vi "GenSet_AE.vi"(7 "Enum":enum16{"READ", "WRITE"}(ring), 10 "General settings":T1={"Holo size (pixels)"=0, "Top hat radius"=0.5, "Number of modes"=0, "Bkg gradient X"=0.0, "Bkg gradient Y"=0.0, "Flat"=FALSE, "Mode Matrix"=0}) -> (2 "General settings Out":T1={"Holo size (pixels)"=0, "Top hat radius"=0.0, "Number of modes"=0, "Bkg gradient X"=0.0, "Bkg gradient Y"=-40.0, "Flat"=FALSE, "Mode Matrix"=0})   [LabVIEW 2014]
uses:
  Controls/SLM General Settings.ctl
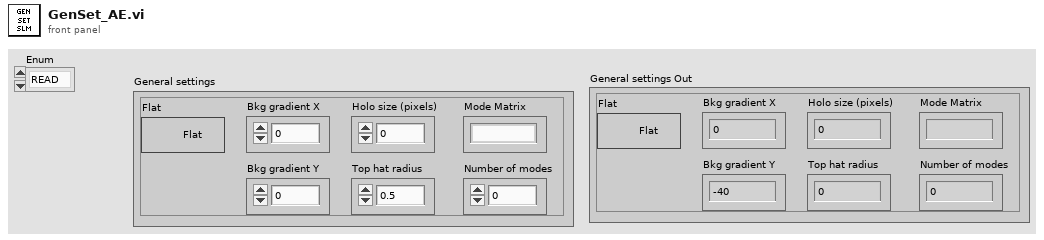
[diagram p1: front panel]
types:
  T1 = typedef "SLM General Settings.ctl" = cluster{"Holo size (pixels)":i32, "Top hat radius":dbl, "Number of modes":i32, "Bkg gradient X":dbl, "Bkg gradient Y":dbl, "Flat":bool, "Mode Matrix":u16}
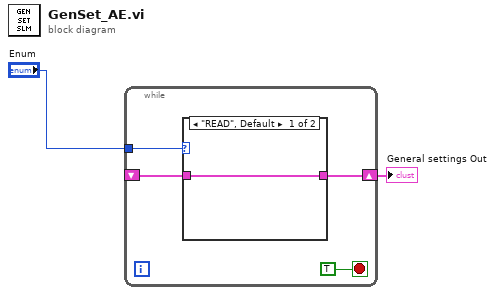
[diagram p0: block diagram]
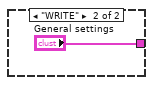
[diagram p2: hidden frame]
diagram:
  n1 = while {
    shift-right: [w5] -> w1
    shift-left: _ -> [w3]
    tunnel: "Enum" -> [w4]
    stop <- TRUE stop-if-true
    n2 = case shown="\"READ\", Default" w4 {
      tunnel: [w7 "General settings"] -> w5
      tunnel: w3 -> [w7 _]
      frame "READ", Default {
      }
      frame "WRITE" {
      }
    }
  }
  "General settings Out" <- w1
